vi "construct_transceive.vi"(0 "burst_mode":enum16{"burst", "continuous"}(ring), 5 "acq_length":i32, 7 "Waveform in":csg[](array[numeric]), 11 "error in (no error) 2":errorcluster) -> (4 "command out":T1=enum."configure_rf", 6 "parameters JSON":string, 10 "data out":variant, 14 "Debug info":string, 15 "error out 2":errorcluster)   [LabVIEW 2019, in "mmW_commands.lvlib"]
uses:
  mmW_commands.lvlib
  <vilib>/addons/_JKI.lib/Serialization/JSON/JKI JSON Serialization.lvlib
  TypeDefs/_depr_datatypes.ctl
  TypeDefs/commands.ctl
  transceive_typedef.ctl
panel:
  out "datatype (only for debug)":T2
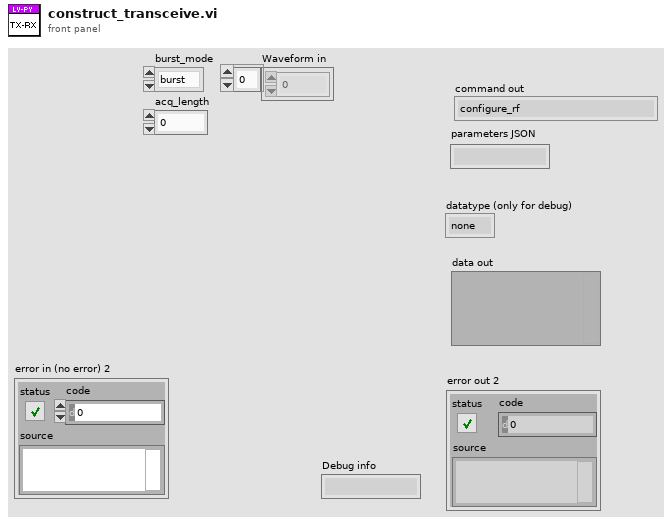
[diagram p1: front panel]
types:
  T1 = typedef "mmW_commands.lvlib/commands.ctl" = enum16{"configure_fs", "configure_rf", "configure_trigger", "equalization_enable", "equalization_start", "lo_sync_enable", "equalization_stop", "get_instrument_status", "get_versions", "initialize_hw", "pop_rx", "set_log_level", "Shutdown", "start", "start_instrument_app", "stop", "trans", "transceive", "trigger_burst", "trigger_sync_enable", "Write TX", "resp_generic", "resp_waveform", "send_trigger", "fetch", "transceive2"}
  T2 = typedef "mmW_commands.lvlib/_depr_datatypes.ctl" = enum16{"none", "float", "string", "CSG_wfm", "DBL_wfm"}
  T3 = typedef "mmW_commands.lvlib/transceive_typedef.ctl" = cluster{"burst_mode":enum16{"burst", "continuous"}, "datatype":string, "acq_length":i32}
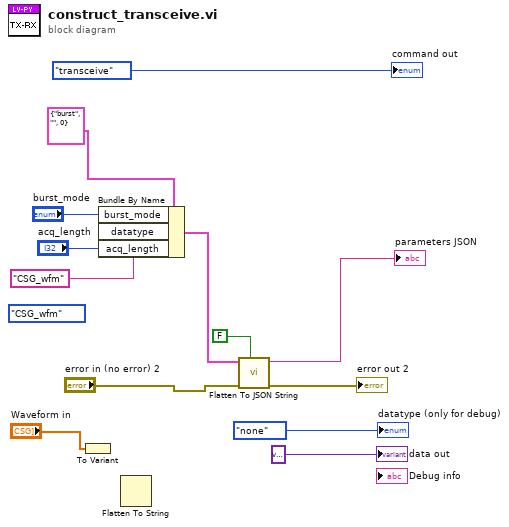
[diagram p0: block diagram]
diagram:
  (unwired) _depr_datatypes."CSG_wfm" ("datatypes")
  n1 = To Variant(anything="Waveform in") -> ()  [unwired: 1 out]
  n2 = Bundle By Name(cluster=T3 {"burst_mode"=enum."burst", "datatype"="", "acq_length"=0} ("Cluster"), "burst_mode"="burst_mode", "datatype"="CSG_wfm", "acq_length"="acq_length") -> (w12:T3)
  n3 = Flatten To String() -> ()  [unwired: 4 in, 3 out]
  n4 = call <vilib>:"Flatten To JSON String.vi"("Multiline (T)"=FALSE, "error in (no error)"="error in (no error) 2", "Variant"=w12) -> ("error out"=→"error out 2":errorcluster, "JSON String"=→"parameters JSON":string)  [unwired: 7 in]
  "datatype (only for debug)" <- _depr_datatypes."none" ("datatypes")
  "data out" <- variant
  "command out" <- commands."transceive" ("mmW_instrument_commands")
